vi "24HP_Parse status bits.vi"(1 "Status bytes":u8[](array[numeric])) -> (0 "Sensor status":bool[][][](array[boolean]))   [LabVIEW 2020]
panel:
  # "bank"
  # "Power"
  # "!Busy"
  # "!MemErr"
  # "!MathSat"
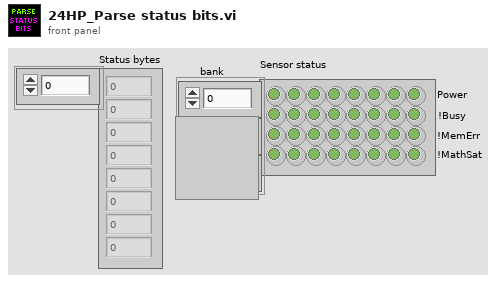
[diagram p1: front panel]
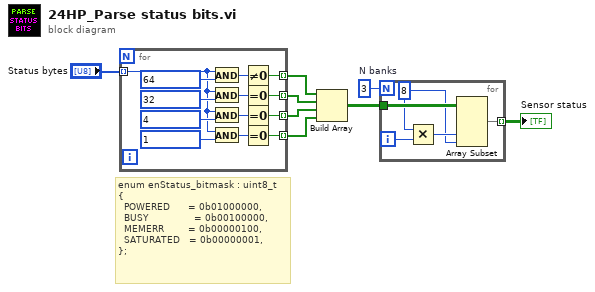
[diagram p0: block diagram]
diagram:
  w3 = 3  # N banks
  # "enum enStatus_bitmask : uint8_t\n{\n  POWERED      = 0b01000000,\n  BUSY               = 0b00100000,\n  MEMERR        = 0b00000100,\n  SATURATED   = 0b00000001,\n};"
  n1 = for {
    tunnel: "Status bytes" -> [w17] mode=indexing
    tunnel: [w9] -> w8 mode=indexing
    tunnel: [w15] -> w7 mode=indexing
    tunnel: [w13] -> w6 mode=indexing
    tunnel: [w11] -> w5 mode=indexing
    n2 = And(x=w17, y=u8 64) -> (x .and. y?=w10:u8)
    n3 = And(x=w17, y=u8 32) -> (x .and. y?=w16:u8)
    n4 = And(x=w17, y=u8 4) -> (x .and. y?=w14:u8)
    n5 = And(x=w17, y=u8 1) -> (x .and. y?=w12:u8)
    n6 = Not Equal To 0?(x=w10) -> (x != 0?=w9:bool)
    n7 = Equal To 0?(x=w16) -> (x = 0?=w15:bool)
    n8 = Equal To 0?(x=w14) -> (x = 0?=w13:bool)
    n9 = Equal To 0?(x=w12) -> (x = 0?=w11:bool)
  }
  n10 = Build Array(w8, w7, w6, w5) -> (w2:bool[][])
  n11 = for {
    N: w3 -> [_]
    tunnel: w2 -> [w26]
    tunnel: [w24] -> w1 mode=indexing
    i -> [w25]
    w22 = 8 ("x")
    n12 = Multiply(x=w22, y=w25) -> (x*y=w23:i32)
    n13 = Array Subset(array=w26, index (col)=w23, length (col)=w22) -> (w24:bool[][])  [unwired: 2 in]
  }
  "Sensor status" <- w1
